vi "CleanupTraces.vi"(8 "Baseline Rate":dbl=0.001, 9 "Spacing":dbl=100.0, 10 "decimating factor":i32=10, 11 "Traces in":waveform(i32)[](array[waveform])) -> (3 "Traces out":waveform(dbl)[](array[waveform]))   [LabVIEW 2014]
uses:
  <vilib>/Analysis/baseanly.llb/Mean (DBL).vi
  <vilib>/Analysis/2dsp.llb/Decimate (continuous, DBL).vi
  <vilib>/Analysis/NI_AALPro.lvlib
  <vilib>/Analysis/NI_AALBase.lvlib
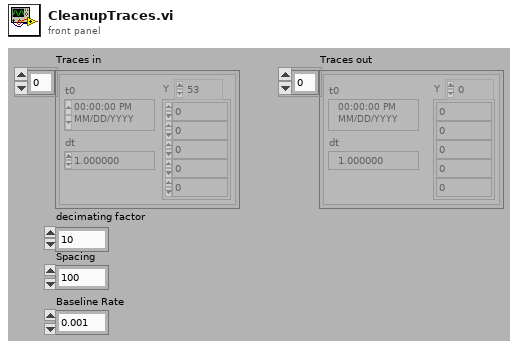
[diagram p1: front panel]
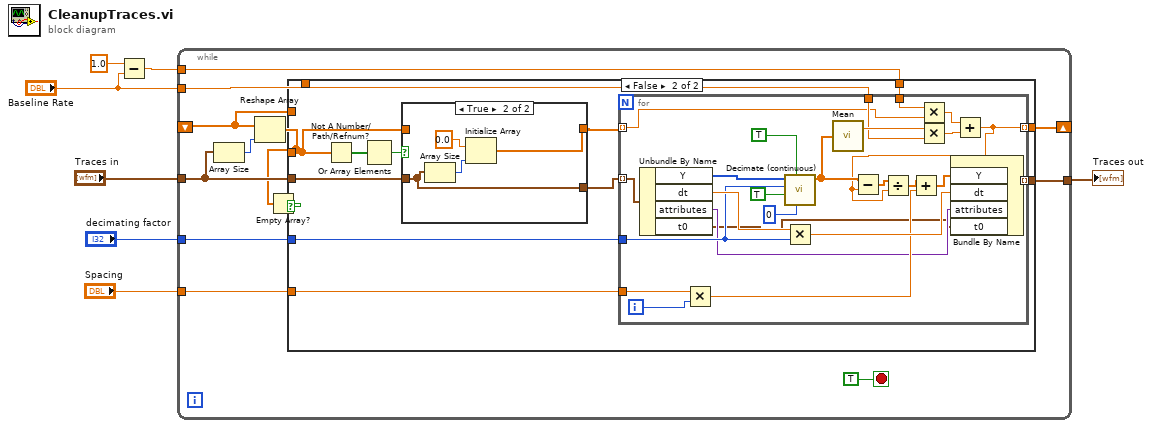
[diagram p0: block diagram]
diagram:
  n1 = Subtract(x=1.0, y="Baseline Rate") -> (x-y=w1:dbl)
  n2 = while {
    tunnel: "Traces in" -> [w12]
    tunnel: "decimating factor" -> [w19]
    tunnel: "Spacing" -> [w18]
    tunnel: [w17] -> w4
    shift-right: [w16] -> _
    shift-left: _ -> [w9]
    tunnel: "Baseline Rate" -> [w14]
    tunnel: w1 -> [w13]
    stop <- TRUE stop-if-true
    n3 = Array Size(array=w12) -> (size(s)=w15:i32)
    n4 = Reshape Array(w9, w15) -> (w11:dbl[])
    n5 = Empty Array?(array=w11) -> (empty?=w10:bool)
    n6 = case shown="False" w10 {
      tunnel: w19 -> [_ w33]
      tunnel: w18 -> [_ w32]
      tunnel: [w20 w31] -> w17
      tunnel: [w21 w30] -> w16
      tunnel: w14 -> [_ w29]
      tunnel: w13 -> [_ w28]
      tunnel: w12 -> [w20 w25]
      tunnel: w11 -> [_ w22]
      tunnel: w9 -> [w21 _]
      frame True {
      }
      frame False {
        n7 = Not A Number/Path/Refnum?(number/path/refnum=w22) -> (NaN/Path/Refnum?=w27:bool[])
        n8 = Or Array Elements(Boolean array=w27) -> (logical OR=w26:bool)
        n9 = case shown="True" w26 {
          tunnel: w25 -> [w34 w39]
          tunnel: [w34 w39] -> w24
          tunnel: [w35 w36] -> w23
          tunnel: w22 -> [w35 _]
          frame False {
          }
          frame True {
            n10 = Array Size(array=w39) -> (size(s)=w38:i32)
            n11 = Initialize Array(0.0, w38) -> (w36:dbl[])
          }
        }
        n12 = for {
          tunnel: w24 -> [w64] mode=indexing
          tunnel: w33 -> [w59]
          tunnel: w32 -> [w56]
          tunnel: [w53] -> w31 mode=indexing
          tunnel: [w40] -> w30 mode=indexing
          tunnel: w23 -> [w44] mode=indexing
          tunnel: w29 -> [w47]
          tunnel: w28 -> [w46]
          i -> [w57]
          n13 = Unbundle By Name(w64) -> ("Y"=w63:i32[], "dt"=w60:dbl, "attributes"=w42:variant, "t0"=w41:timestamp)
          n14 = Multiply(x=w56, y=w57) -> (x*y=w54:dbl)
          n15 = call-poly <vilib>:"Decimate (continuous).vi"("start index"=0, "reset"=TRUE, "averaging"=TRUE, "decimating factor"=w59, "X"=w63) -> ("Decimated Array"=w49:dbl[])  [unwired: 5 in, 1 out]
          n16 = Multiply(x=w60, y=w59) -> (x*y=w58:dbl)
          n17 = call-poly <vilib>:"Mean.vi"("X"=w49) -> ("mean"=w52:dbl)  [unwired: 1 out]
          n18 = Multiply(x=w46, y=w44) -> (x*y=w50:dbl)
          n19 = Multiply(x=w52, y=w47) -> (x*y=w51:dbl)
          n20 = Add(x=w50, y=w51) -> (x+y=w40:dbl)
          n21 = Subtract(x=w49, y=w40) -> (x-y=w45:dbl[])
          n22 = Divide(x=w45, y=w40) -> (x/y=w43:dbl[])
          n23 = Add(x=w43, y=w54) -> (x+y=w55:dbl[])
          n24 = Bundle By Name("Y"=w55, "dt"=w58, "attributes"=w42, "t0"=w41) -> (w53:waveform(dbl))  [unwired: 1 in]
        }
      }
    }
  }
  "Traces out" <- w4
